vi "CreateAndCopyAliasesFile.vi"(9 "IPAddress":string, 10 "TS Bin Path":path=path "C:/Program Files/National Instruments/TestStand 3.5/Bin", 11 "LVDir Path":path=path "D:/LVDev/Saturn/dist") -> (0 "error out":errorcluster)   [LabVIEW 2012]
uses:
  <vilib>/Utility/config.llb/Write Key (String).vi
  <vilib>/Utility/config.llb/NI_LVConfig.lvlib
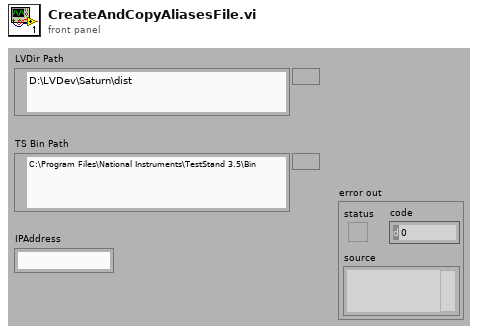
[diagram p1: front panel]
types:
  T1 = typedef "NI_LVConfig.lvlib/Config Data RefNum.ctl" = refnum<k1>
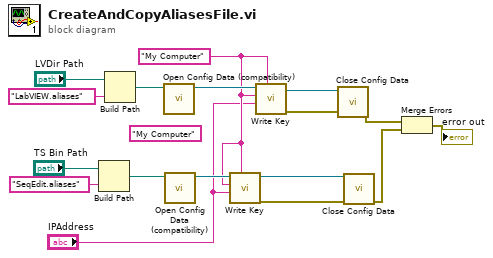
[diagram p0: block diagram]
diagram:
  (unwired) "My Computer" ("section")
  w9 = "My Computer" ("section")
  n1 = Build Path(base path="TS Bin Path", name or relative path="SeqEdit.aliases") -> (appended path=w12:path)
  n2 = Build Path(base path="LVDir Path", name or relative path="LabVIEW.aliases") -> (appended path=w13:path)
  n3 = call <vilib>:"Open Config Data (compatibility).vi"("configuration file path"=w13) -> ("refnum"=w11:T1)  [unwired: 8 in, 2 out]
  n4 = call <vilib>:"Open Config Data (compatibility).vi"("configuration file path"=w12) -> ("refnum"=w10:T1)  [unwired: 8 in, 2 out]
  n5 = call-poly <vilib>:"Write Key.vi"("section"=w9, "value"="IPAddress", "key"=w9, "refnum"=w10) -> ("error out"=w4:errorcluster, "refnum out"=w5:T1)  [unwired: 2 in, 4 out]
  n6 = call-poly <vilib>:"Write Key.vi"("section"=w9, "value"="IPAddress", "key"=w9, "refnum"=w11) -> ("error out"=w6:errorcluster, "refnum out"=w7:T1)  [unwired: 2 in, 4 out]
  n7 = call <vilib>:"Close Config Data.vi"("error in (no error)"=w6, "refnum"=w7) -> ("error out"=w3:errorcluster)  [unwired: 1 in, 8 out]
  n8 = call <vilib>:"Close Config Data.vi"("error in (no error)"=w4, "refnum"=w5) -> ("error out"=w2:errorcluster)  [unwired: 1 in, 8 out]
  n9 = Merge Errors(w3, w2) -> (→"error out":errorcluster)
